vi "Remove Extra Blines.vi"(5 "Z size (pxl)":i32=400, 7 "Data In":u16[][](array[numeric]), 9 "#Aline":i32=400, 10 "Start index":i32, 11 "nAT per B":i32) -> (6 "Data Out":u16[][](array[numeric]))   [LabVIEW 2017]
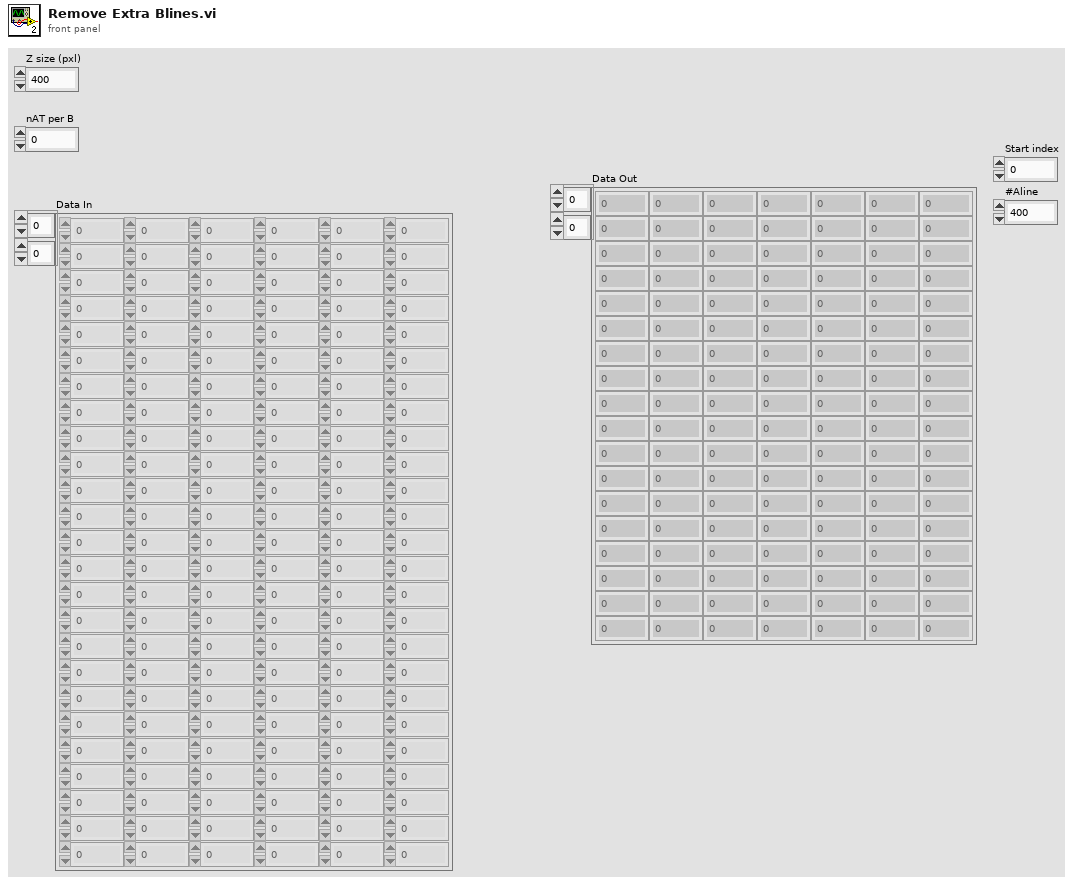
[diagram p1: front panel]
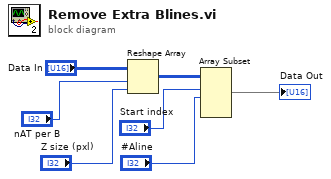
[diagram p0: block diagram]
diagram:
  n1 = Reshape Array("Data In", "nAT per B", "Z size (pxl)") -> (w5:u16[][])
  n2 = Array Subset(array=w5, index (row)="Start index", length (row)="#Aline") -> (→"Data Out":u16[][])  [unwired: 2 in]
